vi "RIO 7961R (FPGA).vi"() -> ()   [LabVIEW 2016]
doc: "This FPGA VI transfers data samples to the host using a stream. The stream is controlled from the host."
uses:
  <vilib>/Platform/TimedLoop/XDataNode/timing_clust.ctl
  <vilib>/Platform/TimedLoop/XDataNode/nitl_modes.ctl
  <vilib>/Platform/TimedLoop/XDataNode/wakeup.ctl
  <vilib>/rvi/Emulation/niFpgaGetClockAttributes.vi
  <vilib>/rvi/Emulation/niFpgaSctlEmulationGetInTimedLoop.vi
  <vilib>/rvi/Emulation/niFpgaEmulationReportErrorSimple.vi
  <vilib>/rvi/eio/common/nirviEmuTemplateMethod_errors.vi
  <vilib>/rvi/Emulation/niFpgaCriticalErrorInLSC.vi
  <vilib>/rvi/interface/RandomDataEmulation/niFpgaRandomDataHandleErrors.vi
  <vilib>/eio/EIONode/EIONode.xnode
  <vilib>/Platform/TimedLoop/XDataNode/XDataNode.xnode
  <vilib>/rvi/DataTransferAndStorage/Container/XNode/niFpgaContainer.xnode
  <vilib>/rvi/interface/RandomDataEmulation/nirviRandomDataFpgaReadWriteTemplate.vi
  <vilib>/Platform/TimedLoop/XDataNode/XDNodeRunTimeDep.lvlib
panel:
  in  "Gain":u8(ring)=1 items=["12 db"=2, "6 db"=1, "0 db"=0]
  in  "Coupling":u8(ring)=1 items=["DC"=1, "AC"=0]
  out "IO Module\\Initialization Done":bool
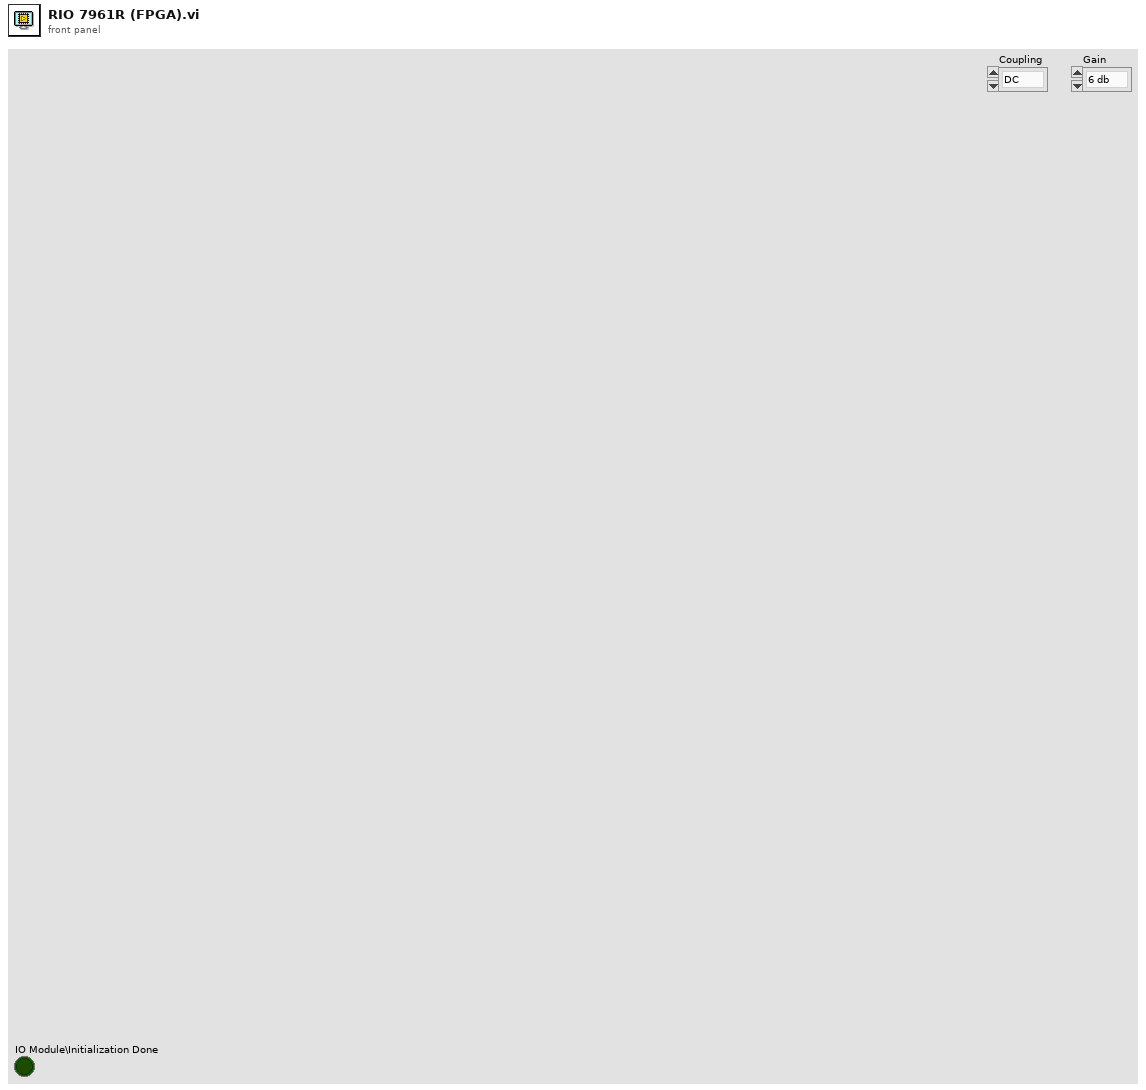
[diagram p1: front panel]
types:
  T1 = typedef "XDNodeRunTimeDep.lvlib/timing_clust.ctl" = cluster{"Expected End [f-1]":u64, "Actual End [f-1]":u64, "Finished Late? [f-1]":bool, "Expected End [i-1]":u64, "Actual End [i-1]":u64, "Finished Late? [i-1]":bool, "Expected Start [i]":u64, "Actual Start [i]":u64, "Expected Start [f]":u64, "Actual Start [f]":u64, "Source Name":string, "Structure Name":string, "Period":i64, "Deadline":i64, "Offset":i64, "Start":i64, "Priority":i32, "Timeout":i32, "Mode":T2, "Wakeup Reason":T3, "Error":errorcluster, "Source Type":string, "Secondary Source Type":string, "Global End Time":u64, "Global Start Time":u64, "Frame Duration":u64, "Iteration Duration":u64, "Assigned CPU":i32, "I/O Scan Engine Mode":u32}
  T2 = typedef "XDNodeRunTimeDep.lvlib/nitl_modes.ctl" = enum32{"No Change", "Process missed periods, maintain original phase", "Discard missed periods, maintain original phase", "Process missed periods, ignore original phase", "Discard missed periods, ignore original phase"}
  T3 = typedef "XDNodeRunTimeDep.lvlib/wakeup.ctl" = enum32{"Normal", "Aborted", "Asynchronous wakeup", "Timing source error", "Timed loop error", "Timeout"}
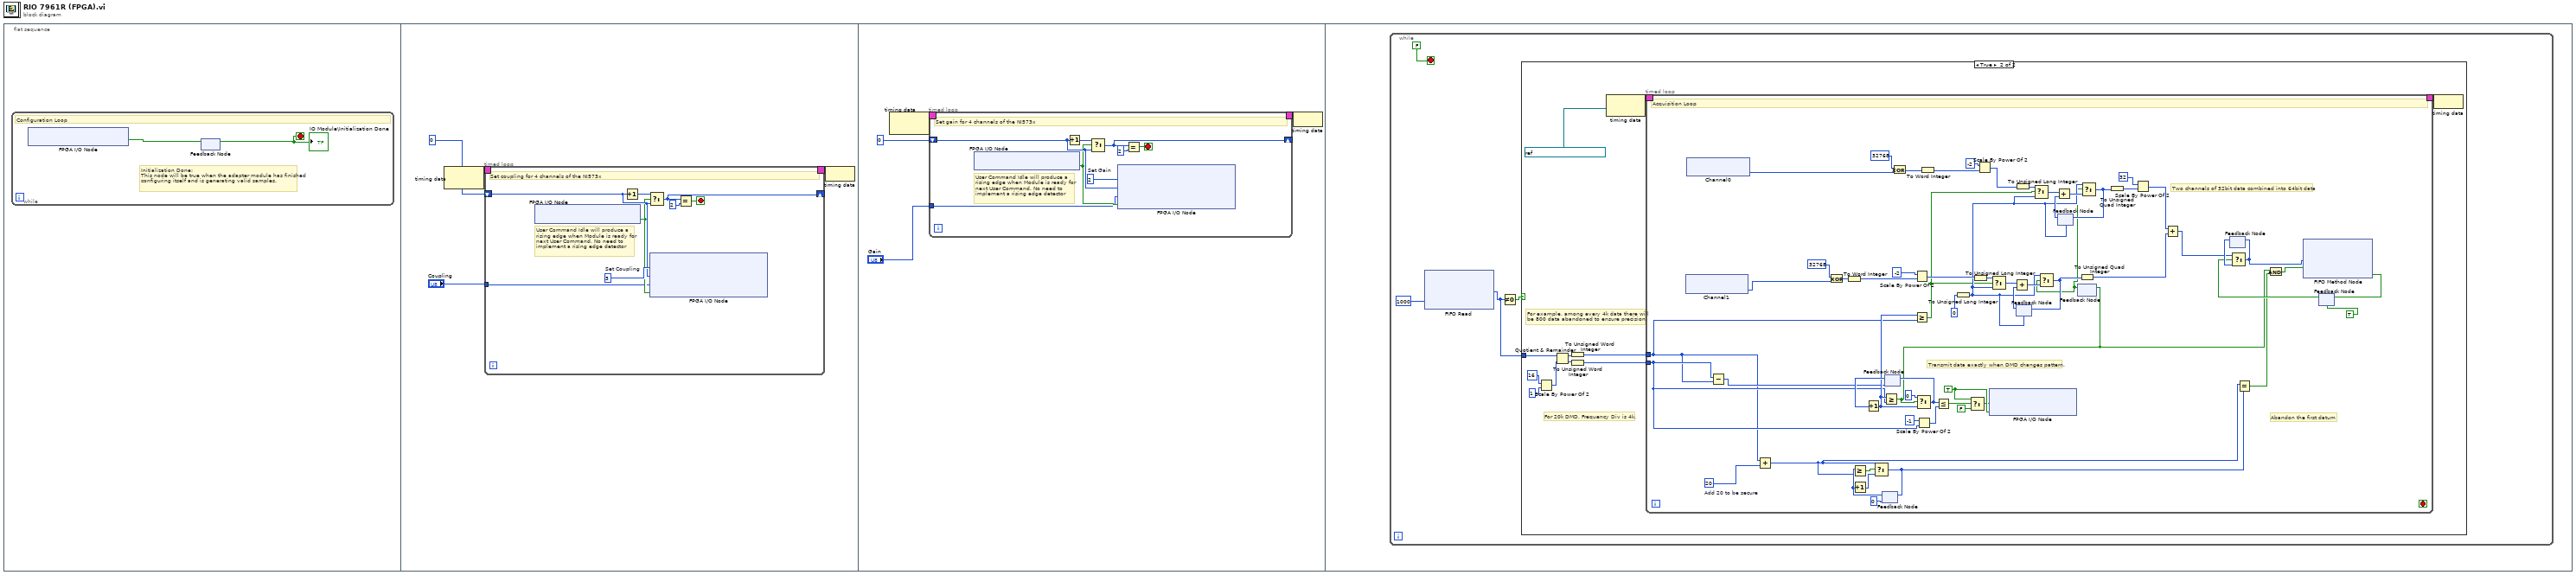
[diagram p0: block diagram]
diagram:
  n1 = flat-sequence {
    frame #0 {
      n2 = while {
        stop <- w1 stop-if-true
        # "Initialization Done:\nThis node will be true when the adapter module has finished configuring itself and is generating valid samples."
        # "Configuration Loop"
        n3 = xnode "FPGA I/O Node"() -> ("IO Module\\Initialization Done"=w2:bool)  [unwired: 1 in, 1 out]
        n4 = feedback-in #1(w2) -> ()
        n5 = feedback #1() -> (w1:bool)  [unwired: 1 in]
        "IO Module\\Initialization Done" <- w1
      }
    }
    frame #1 {
      n6 = node-c288() -> (w6:T1)  [unwired: 1 in]
      n7 = timed-loop {
        timing: w6 -> [_]
        timing-out: [_] -> w5
        shift-right: [w9] -> _
        shift-left: u8 0 -> [w10]
        tunnel: "Coupling" -> [w7]
        stop <- w12 stop-if-true
        w14 = u8 3  # Set Coupling
        # "User Command Idle will produce a\nrising edge when Module is ready for\nnext User Command. No need to\nimplement a rising edge detector"
        # "Set coupling for 4 channels of the NI573x"
        n8 = xnode "FPGA I/O Node"() -> ("IO Module\\User Command Idle"=w8:bool)  [unwired: 1 in, 1 out]
        n9 = Increment(x=w10) -> (x+1=w11:u8)
        n10 = Select(t=w11, s=w8, f=w10) -> (s? t:f=w9:u8)
        n11 = xnode ("FPGA I/O Node")("IO Module\\User Command"=w14, "IO Module\\User Data 0"=w10, "IO Module\\User Data 1"=w7, "IO Module\\User Command Commit"=w8) -> ()  [unwired: 4 in, 4 out]
        n12 = Equal?(x=w9, y=u8 2) -> (x = y?=w12:bool)
      }
      n13 = node-c288(w5) -> ()
    }
    frame #2 {
      n14 = node-c288() -> (w22:T1)  [unwired: 1 in]
      n15 = timed-loop {
        timing: w22 -> [_]
        timing-out: [_] -> w21
        shift-right: [w25] -> _
        shift-left: u8 0 -> [w26]
        tunnel: "Gain" -> [w23]
        stop <- w28 stop-if-true
        w30 = u8 2  # Set Gain
        # "User Command Idle will produce a\nrising edge when Module is ready for\nnext User Command. No need to\nimplement a rising edge detector"
        # "Set gain for 4 channels of the NI573x"
        n16 = xnode "FPGA I/O Node"() -> ("IO Module\\User Command Idle"=w24:bool)  [unwired: 1 in, 1 out]
        n17 = Increment(x=w26) -> (x+1=w27:u8)
        n18 = Select(t=w27, s=w24, f=w26) -> (s? t:f=w25:u8)
        n19 = xnode ("FPGA I/O Node")("IO Module\\User Command"=w30, "IO Module\\User Data 0"=w26, "IO Module\\User Data 1"=w23, "IO Module\\User Command Commit"=w24) -> ()  [unwired: 4 in, 4 out]
        n20 = Equal?(x=w25, y=u8 2) -> (x = y?=w28:bool)
      }
      n21 = node-c288(w21) -> ()
    }
    frame #3 {
      n22 = while {
        stop <- FALSE stop-if-true
        n23 = xnode "FIFO Read"("Timeout"=1000) -> ("Element"=w35:u32)  [unwired: 1 in, 2 out]
        n24 = Not Equal To 0?(x=w35) -> (x != 0?=w36:bool)
        n25 = case shown="True" w36 {
          tunnel: w35 -> [_ w46]
          frame False {
          }
          frame True {
            # "For example, among every 4k data there will \nbe 800 data abandoned to ensure precision."
            # "For 20k DMD, Frequency Div is 4k."
            n26 = Scale By Power Of 2(n=i16 16, x=u32 1) -> (x*2^n=w43:u32)
            n27 = Quotient & Remainder(x=w46, y=w43) -> (x-y*floor(x/y)=w41:u32, floor(x/y)=w42:u32)
            n28 = To Unsigned Word Integer(number=w41) -> (unsigned 16bit integer=w40:u16)
            n29 = To Unsigned Word Integer(number=w42) -> (unsigned 16bit integer=w39:u16)
            n30 = node-c288(refnum<k21> "IO Module\\Sample Clock" ("Source Name")) -> (w49:T1)
            n31 = timed-loop {
              timing: w49 -> [_]
              timing-out: [_] -> w48
              tunnel: w40 -> [w50]
              tunnel: w39 -> [w55]
              stop <- _ stop-if-true
              w62 = u16 20  # Add 20 to be secure
              w103 = TRUE
              # "Two channels of 32bit data combined into 64bit data"
              # "Transmit data exactly when DMD changes pattern."
              # "Abandon the first datum"
              # "Acquisition Loop"
              n32 = xnode "Channel1"() -> ("IO Module\\AI 1"=w79:u16)  [unwired: 1 in, 1 out]
              n33 = xnode "Channel0"() -> ("IO Module\\AI 0"=w106:u16)  [unwired: 1 in, 1 out]
              n34 = Subtract(x=w55, y=w50) -> (x-y=w56:u16)
              n35 = Add(x=w50, y=w62) -> (x+y=w57:u16)
              n36 = Exclusive Or(1:w79, 2:u16 32768 ("x")) -> (0:w80:u16)
              n37 = To Word Integer(number=w80) -> (16bit integer=w82:i16)
              n38 = feedback #2(u16 0) -> (w60:u16)
              n39 = Greater Or Equal?(x=w60, y=w57) -> (x >= y?=w61:bool)
              n40 = Increment(x=w60) -> (x+1=w59:u16)
              n41 = Select(t=w57, s=w61, f=w59) -> (s? t:f=w58:u16)
              n42 = feedback-in #2(w58) -> ()
              n43 = feedback #3(w56) -> (w99:u16)
              n44 = Increment(x=w99) -> (x+1=w87:u16)
              n45 = Greater Or Equal?(x=w87, y=w55) -> (x >= y?=w71:bool)
              n46 = Exclusive Or(1:w106, 2:u16 32768 ("x")) -> (0:w104:u16)
              n47 = Scale By Power Of 2(n=i16 -2, x=w82) -> (x*2^n=w73:i16)
              n48 = Greater Or Equal?(x=w87, y=w50) -> (x >= y?=w52:bool)
              n49 = Select(t=u16 0, s=w71, f=w87) -> (s? t:f=w97:u16)
              n50 = feedback-in #3(w97) -> ()
              n51 = Scale By Power Of 2(n=i16 -1, x=w55) -> (x*2^n=w53:u16)
              n52 = To Word Integer(number=w104) -> (16bit integer=w107:i16)
              n53 = Less Or Equal?(x=w97, y=w53) -> (x <= y?=w100:bool)
              n54 = To Unsigned Long Integer(number=i16 0 ("f")) -> (unsigned 32bit integer=w72:u32)
              n55 = Select(t=w103, s=w100, f=FALSE) -> (s? t:f=w102:bool)
              n56 = To Unsigned Long Integer(number=w73) -> (unsigned 32bit integer=w77:u32)
              n57 = Scale By Power Of 2(n=i16 -2, x=w107) -> (x*2^n=w86:i16)
              n58 = xnode "FPGA I/O Node"("IO Module\\PFI 0 Wr Data"=w102, "IO Module\\PFI 0 WE"=w103) -> ()  [unwired: 2 in, 2 out]
              n59 = Select(t=w77, s=w52, f=w72) -> (s? t:f=w74:u32)
              n60 = To Unsigned Long Integer(number=w86) -> (unsigned 32bit integer=w91:u32)
              n61 = feedback #4(w72) -> (w76:u32)
              n62 = Add(x=w74, y=w76) -> (x+y=w75:u32)
              n63 = Select(t=w91, s=w52, f=w72) -> (s? t:f=w88:u32)
              n64 = feedback #5(w72) -> (w90:u32)
              n65 = Add(x=w88, y=w90) -> (x+y=w89:u32)
              n66 = feedback #6() -> (w51:bool)  [unwired: 1 in]
              n67 = Select(t=w72, s=w51, f=w75) -> (s? t:f=w66:u32)
              n68 = feedback-in #4(w66) -> ()
              n69 = feedback-in #6(w71) -> ()
              n70 = To Unsigned Quad Integer(1:w66) -> (0:w65:u64)
              n71 = Select(t=w72, s=w51, f=w89) -> (s? t:f=w70:u32)
              n72 = feedback-in #5(w70) -> ()
              n73 = To Unsigned Quad Integer(1:w70) -> (0:w69:u64)
              n74 = Scale By Power Of 2(n=i16 32, x=w69) -> (x*2^n=w67:u64)
              n75 = Add(x=w67, y=w65) -> (x+y=w64:u64)
              n76 = feedback #7() -> (w95:u64)  [unwired: 1 in]
              n77 = Equal?(x=w57, y=w58) -> (x = y?=w85:bool)
              n78 = And(x=w71, y=w85) -> (x .and. y?=w84:bool)
              n79 = feedback #8(TRUE) -> (w94:bool)
              n80 = Select(t=w64, s=w94, f=w95) -> (s? t:f=w92:u64)
              n81 = feedback-in #7(w92) -> ()
              n82 = xnode ("FIFO Method Node")("Element"=w92, "Input Valid"=w84) -> ("Ready for Input"=w93:bool)  [unwired: 1 in, 1 out]
              n83 = feedback-in #8(w93) -> ()
            }
            n84 = node-c288(w48) -> ()
          }
        }
      }
    }
  }
